vi "Read Stored State DVR.vi"(8 "error in (no error)":errorcluster, 11 "Cal Sequence Builder in":refnum<class "Cal Sequence Builder.lvclass">) -> (0 "error out":errorcluster, 2 "Stored State DVR":refnum<data-value>, 3 "Cal Sequence Builder out":refnum<class "Cal Sequence Builder.lvclass">)   [LabVIEW 2015, in "Cal Sequence Builder.lvclass"]
uses:
  Cal Sequence Builder.lvclass
  State data/State Data.lvclass
  Cal Sequence Builder.lvclass/Cal Sequence Builder.ctl
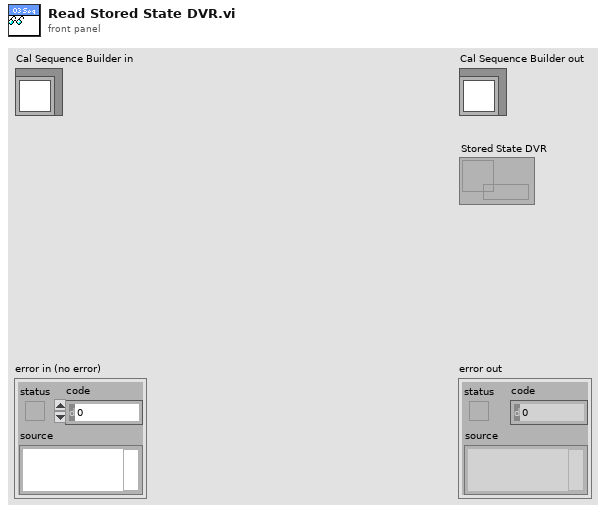
[diagram p1: front panel]
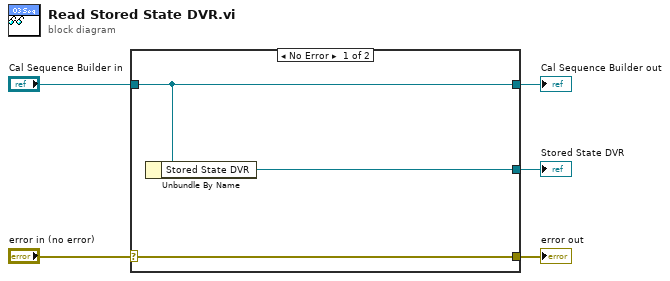
[diagram p0: block diagram]
diagram:
  n1 = case shown="No Error" "error in (no error)" {
    selector: "error in (no error)" -> [w8 w9]
    tunnel: [w8 w9] -> w4
    tunnel: [w7 w10] -> w2
    tunnel: "Cal Sequence Builder in" -> [w7 w10]
    tunnel: [w6 _] -> w1
    frame No Error {
      n2 = Unbundle By Name(w7) -> ("Stored State DVR"=w6:refnum<data-value>)
    }
    frame Error {
    }
  }
  "error out" <- w4
  "Cal Sequence Builder out" <- w2
  "Stored State DVR" <- w1
